vi "更新程序.vi"   [LabVIEW 2017]
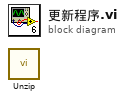
[diagram p0: block diagram]
diagram:
  n1 = call "Unzip.vi"() -> ()  [unwired: 12 in]
